vi "error_code_print.vi"(8 "error in (no error)":errorcluster, 10 "array":dbl[](array[numeric])) -> (0 "error out":errorcluster, 2 "error our":string)   [LabVIEW 2013]
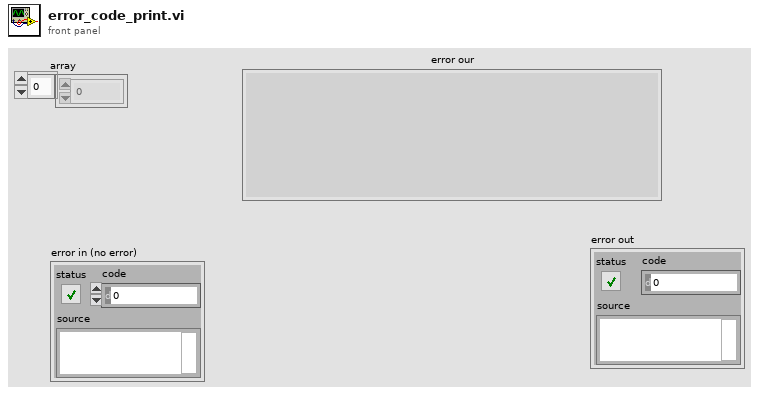
[diagram p1: front panel]
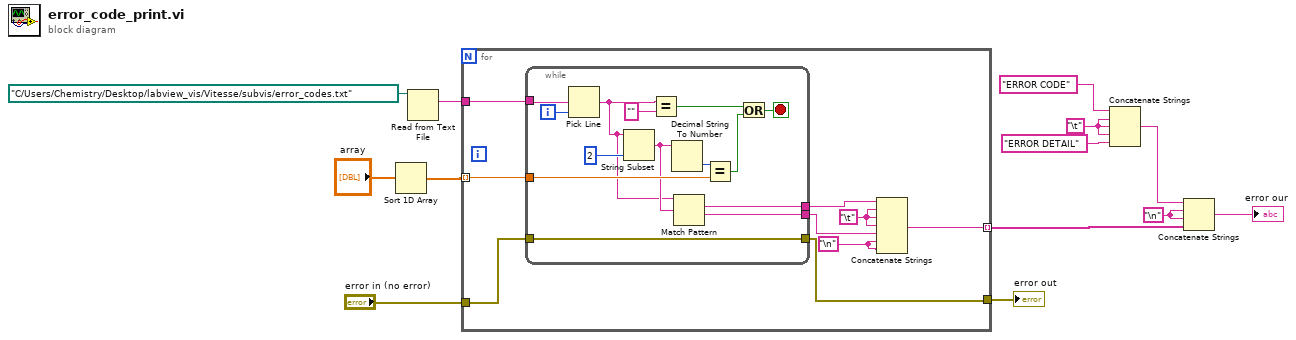
[diagram p0: block diagram]
diagram:
  w4 = "\n"
  w6 = "\t"
  n1 = Sort 1D Array(array="array") -> (sorted array=w8:dbl[])
  n2 = Read from Text File(file (use dialog)=path "C:/Users/Chemistry/Desktop/labview_vis/Vitesse/subvis/error_codes.txt") -> (text=w13:string)  [unwired: 3 in, 3 out]
  n3 = for {
    tunnel: w8 -> [w22] mode=indexing
    tunnel: w13 -> [w21]
    tunnel: [w19] -> w5 mode=indexing
    tunnel: "error in (no error)" -> [w15]
    tunnel: [w14] -> w2
    w16 = "\n"
    w17 = "\t"
    n4 = while {
      tunnel: w21 -> [w36]
      tunnel: w22 -> [w31]
      tunnel: [w26] -> w18
      tunnel: [w25] -> w20
      tunnel: w15 -> [w23]
      tunnel: [w23] -> w14
      i -> [w34]
      stop <- w28 stop-if-true
      n5 = Pick Line(multi-line string=w36, line index=w34) -> (output string=w24:string)  [unwired: 1 in]
      n6 = String Subset(string=w24, length (rest)=2 ("length (rest)")) -> (substring=w27:string)  [unwired: 1 in]
      n7 = Equal?(x=w24, y="") -> (x = y?=w30:bool)
      n8 = Decimal String To Number(string=w27) -> (number=w32:i32)  [unwired: 2 in, 1 out]
      n9 = Match Pattern(string=w24, regular expression=w27) -> (match substring=w25:string, after substring=w26:string)  [unwired: 1 in, 2 out]
      n10 = Equal?(x=w32, y=w31) -> (x = y?=w29:bool)
      n11 = Or(x=w30, y=w29) -> (x .or. y?=w28:bool)
    }
    n12 = Concatenate Strings(w20, w17, w17, w17, w18, w16, w16) -> (w19:string)
  }
  "error out" <- w2
  n13 = Concatenate Strings("ERROR CODE", w6, w6, w6, "ERROR DETAIL") -> (w11:string)
  n14 = Concatenate Strings(w11, w4, w4, w5) -> (→"error our":string)
